vi "ma_sml_Window Frequency Response (first derivative).vi"   [LabVIEW 2020, in "NI_MAPro.lvlib"]
uses:
  NI_MAPro.lvlib
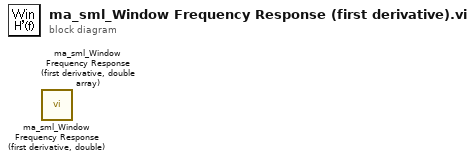
[diagram p0: block diagram]
diagram:
  n1 = call "ma_sml_Window Frequency Response (first derivative, double).vi"() -> ()  [unwired: 3 in, 1 out]
  n2 = call "ma_sml_Window Frequency Response (first derivative, double array).vi"() -> ()  [unwired: 3 in, 1 out]
